vi "toml_remove_key.vi"(4 "vi":refnum<vi>, 7 "section":string, 8 "error in (no error)":errorcluster, 10 "key":string, 11 "path in":path) -> (0 "error out":errorcluster, 2 "key exists":bool, 3 "path out":path)   [LabVIEW 2017]
uses:
  <vilib>/Utility/error.llb/Clear Errors.vi
  toml_lock_obtain.vi
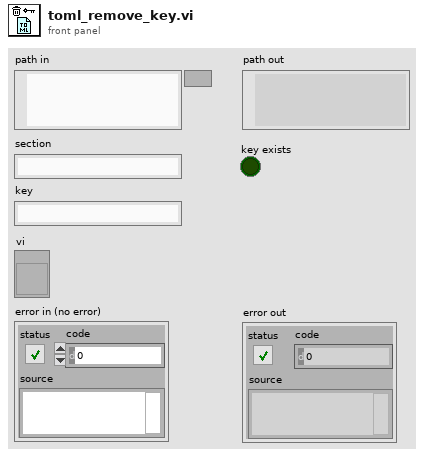
[diagram p1: front panel]
types:
  T1 = enum16{"open", "replace", "create", "open or create", "replace or create", "replace or create with confirmation"}
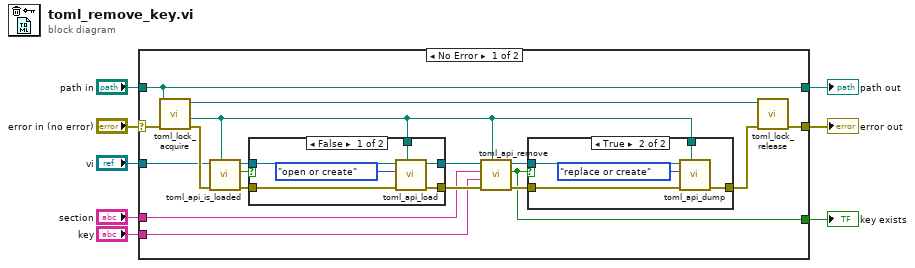
[diagram p0: block diagram]
diagram:
  n1 = case shown="No Error" "error in (no error)" {
    selector: "error in (no error)" -> [w25 w41]
    tunnel: [w24 w41] -> w7
    tunnel: "vi" -> [w18 _]
    tunnel: "path in" -> [w23 w42]
    tunnel: [w23 w42] -> w4
    tunnel: "section" -> [w15 _]
    tunnel: "key" -> [w14 _]
    tunnel: [w9 _] -> w1
    frame No Error {
      n2 = call "toml_lock_acquire.vi"("error in (no error)"=w25, "path in"=w23) -> ("error out"=w19:errorcluster, "resolved path"=w11:path, "lock"=w26:refnum<queue>)  [unwired: 7 in]
      n3 = call "toml_api_is_loaded.vi"("resolved path"=w11, "error in (no error)"=w19, "vi in"=w18) -> ("error out"=w21:errorcluster, "file loaded"=w22:bool, "vi out"=w20:refnum<vi>)  [unwired: 5 in, 1 out]
      n4 = case shown="False" w22 {
        tunnel: w21 -> [w32 w34]
        tunnel: [w31 w34] -> w17
        tunnel: w11 -> [w28 _]
        tunnel: w20 -> [w30 w33]
        tunnel: [w29 w33] -> w16
        frame False {
          n5 = call "toml_api_load.vi"("resolved path"=w28, "error in (no error)"=w32, "operation"=T1."open or create" ("operation (open or create)"), "vi in"=w30) -> ("error out"=w31:errorcluster, "vi out"=w29:refnum<vi>)  [unwired: 5 in, 1 out]
        }
        frame True {
        }
      }
      n6 = call "toml_api_remove.vi"("resolved path"=w11, "error in (no error)"=w17, "key"=w14, "section"=w15, "vi in"=w16) -> ("error out"=w13:errorcluster, "key exists"=w9:bool, "vi out"=w12:refnum<vi>)  [unwired: 4 in]
      n7 = case shown="True" w9 {
        tunnel: w13 -> [w35 w40]
        tunnel: w12 -> [_ w39]
        tunnel: w11 -> [_ w37]
        tunnel: [w35 w36] -> w10
        frame False {
        }
        frame True {
          n8 = call "toml_api_dump.vi"("resolved path"=w37, "error in (no error)"=w40, "operation (open or create)"=T1."replace or create", "vi in"=w39) -> ("error out"=w36:errorcluster)  [unwired: 5 in, 2 out]
        }
      }
      n9 = call "toml_lock_release.vi"("error in (no error)"=w10, "lock"=w26) -> ("error out"=w24:errorcluster)  [unwired: 9 in]
    }
    frame Error {
    }
  }
  "error out" <- w7
  "path out" <- w4
  "key exists" <- w1
